vi "DP-Initialize Run.vi"(5 "Parameters":T1, 7 "acoustic system":string, 11 "error in (no error)":errorcluster) -> (4 "State":T4, 6 "DP Freqs":T5[](array[typedef]), 15 "error out":errorcluster)   [LabVIEW 2020]
uses:
  Typedefs/DP-Freqs.ctl
  Typedefs/DP-Runtime State.ctl
  Typedefs/DP-Parameters.ctl
  Typedefs/DP-Stimulus Params.ctl
  Typedefs/DP-Response Params.ctl
  9b327534-a05b-4f1e-8ea6-4dc0965c4c0a.vi
  53cc11d0-0777-45da-a4da-e21edc2e8946.vi
  0925d4c8-c7d7-466b-8d9d-3b6ad316888a.vi
  <vilib>/Utility/config.llb/Open Config Data.vi
  <vilib>/Utility/config.llb/Get Key Names.vi
  <vilib>/Utility/config.llb/Read Key.vi
  <vilib>/Utility/config.llb/Read Key (String).vi
  epl-vi-lib/Utility VIs/Array Manipulation VIs/String Array to Comma Separated String.vi
  <vilib>/Utility/error.llb/Error Cluster From Error Code.vi
  <vilib>/Utility/config.llb/Close Config Data.vi
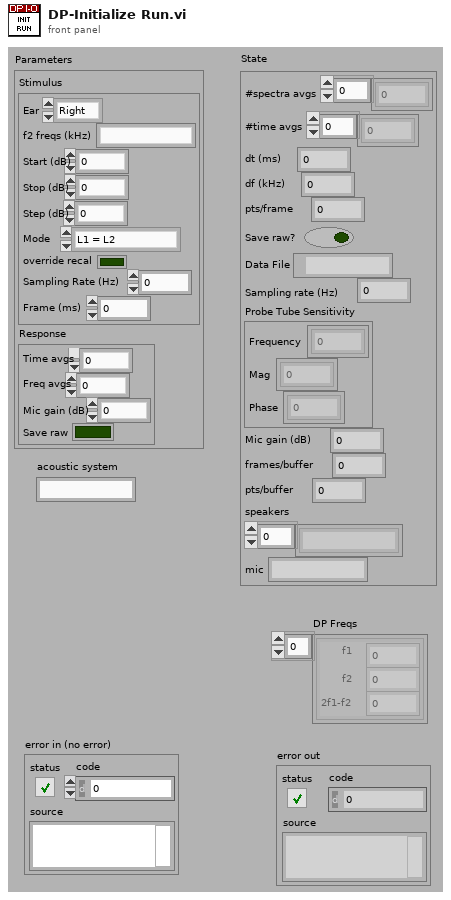
[diagram p1: front panel]
types:
  T1 = typedef "DP-Parameters.ctl" = cluster{"Stimulus":T2, "Response":T3}
  T2 = typedef "DP-Stimulus Params.ctl" = cluster{"Ear":enum16{"Right", "Left"}, "f2 freqs (kHz)":string, "Start (dB)":dbl, "Stop (dB)":dbl, "Step (dB)":dbl, "Mode":enum16{"L1 = L2", "L1 = L2 + 10 dB"}, "override recal":bool, "Sampling Rate (Hz)":dbl, "Frame (ms)":dbl}
  T3 = typedef "DP-Response Params.ctl" = cluster{"Time avgs":i32, "Freq avgs":i32, "Mic gain (dB)":dbl, "Save raw":bool}
  T4 = typedef "DP-Runtime State.ctl" = cluster{"#spectra avgs":i32[], "#time avgs":i32[], "dt (ms)":dbl, "df (kHz)":dbl, "pts/frame":i32, "Save raw?":bool, "Data File":path, "Sampling rate (Hz)":dbl, "Probe Tube Sensitivity":cluster{"Frequency":dbl[], "Mag":dbl[], "Phase":dbl[]}, "Mic gain (dB)":dbl, "frames/buffer":i32, "pts/buffer":i32, "speakers":string[], "mic":string}
  T5 = typedef "DP-Freqs.ctl" = cluster{"f1":dbl, "f2":dbl, "2f1-f2":dbl}
  T6 = cluster{"Coerced Frequency (kHz)":dbl, "Coerced Frequency (kHz)":dbl, dbl}
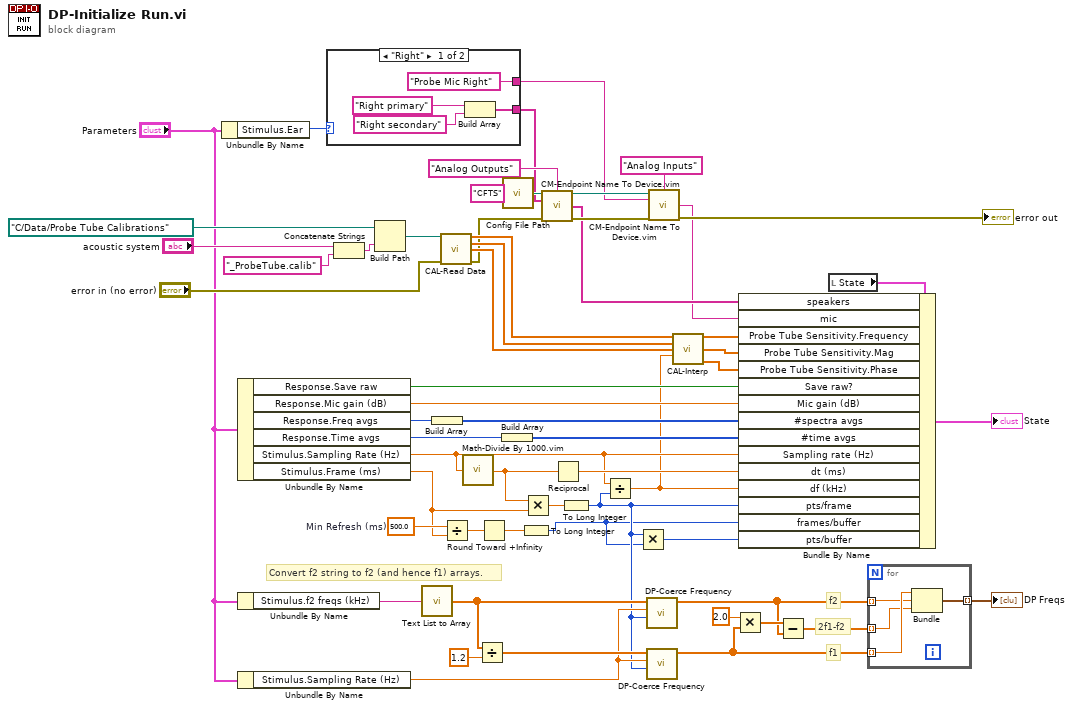
[diagram p0: block diagram]
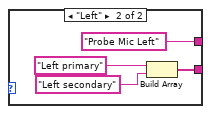
[diagram p2: hidden frame]
diagram:
  w28 = 500.0  # Min Refresh (ms)
  # "2f1-f2"
  # "f2"
  # "f1"
  # "Convert f2 string to f2 (and hence f1) arrays."
  n1 = Unbundle By Name("Parameters") -> ("Stimulus.Ear"=w14:enum16{"Right", "Left"})
  n2 = Unbundle By Name("Parameters") -> ("Response.Save raw"=w33:bool, "Response.Mic gain (dB)"=w34:dbl, "Response.Freq avgs"=w44:i32, "Response.Time avgs"=w43:i32, "Stimulus.Sampling Rate (Hz)"=w30:dbl, "Stimulus.Frame (ms)"=w27:dbl)
  n3 = Unbundle By Name("Parameters") -> ("Stimulus.f2 freqs (kHz)"=w56:string)
  n4 = Unbundle By Name("Parameters") -> ("Stimulus.Sampling Rate (Hz)"=w47:dbl)
  n5 = case shown="\"Right\"" w14 {
    tunnel: [w59 w63] -> w7
    tunnel: ["Probe Mic Right" "Probe Mic Left"] -> w8
    frame "Right" {
      n6 = Build Array("Right primary", "Right secondary") -> (w59:string[])
    }
    frame "Left" {
      n7 = Build Array("Left primary", "Left secondary") -> (w63:string[])
    }
  }
  n8 = Concatenate Strings("acoustic system", "_ProbeTube.calib") -> (w39:string)
  n9 = Build Path(base path=path "C:/Data/Probe Tube Calibrations", name or relative path=w39) -> (appended path=w35:path)
  n10 = call "Text List to Array.vi"("text list"=w56) -> ("array"=w55:dbl[])  [unwired: 3 in]
  n11 = Build Array(w44) -> (w41:i32[])
  n12 = call "CAL-Read Data.vi"("user path"=w35, "error in (no error)"="error in (no error)") -> ("Frequency (Hz)"=w18:dbl[], "Mag"=w17:dbl[], "Phase"=w16:dbl[], "error out"=w4:errorcluster)  [unwired: 9 in, 1 out]
  n13 = Divide(x=w28, y=w27) -> (x/y=w26:dbl)
  n14 = call "Math-Divide By 1000.vim"("X"=w30) -> ("1000X"=w32:dbl)
  n15 = Divide(x=w55, y=1.2) -> (x/y=w54:dbl[])
  n16 = Round Toward +Infinity(x=w26) -> (ceil(x): smallest int >= x=w25:dbl)
  n17 = Build Array(w43) -> (w40:i32[])
  n18 = call "Config File Path.vi"("AppName"="CFTS") -> ("Default config file name"=w12:path)
  n19 = To Long Integer(number=w25) -> (32bit integer=w23:i32)
  n20 = Multiply(x=w32, y=w27) -> (x*y=w31:dbl)
  n21 = call "CM-Endpoint Name To Device.vim"("Path"=w12, "IO Type"="Analog Outputs", "Names in"=w7, "error in (no error)"=w4) -> ("Path thru"=w9:path, "Devices"=w2:string[], "error out"=w6:errorcluster)  [unwired: 8 in, 1 out]
  n22 = Reciprocal(x=w32) -> (1/x=w42:dbl)
  n23 = To Long Integer(number=w31) -> (32bit integer=w24:i32)
  n24 = Divide(x=w30, y=w24) -> (x/y=w15:dbl)
  n25 = Multiply(x=w24, y=w23) -> (x*y=w22:i32)
  n26 = call "DP-Coerce Frequency.vi"("Npts"=w24, "Sampling rate (Hz)"=w47, "Frequency (kHz)"=w55) -> ("Coerced Frequency (kHz)"=w52:dbl[])  [unwired: 6 in, 2 out]
  n27 = call "DP-Coerce Frequency.vi"("Npts"=w24, "Sampling rate (Hz)"=w47, "Frequency (kHz)"=w54) -> ("Coerced Frequency (kHz)"=w50:dbl[])  [unwired: 6 in, 2 out]
  n28 = call "CM-Endpoint Name To Device.vim"("Path"=w9, "IO Type"="Analog Inputs", "Names in"=w8, "error in (no error)"=w6) -> ("Devices"=w1:string, "error out"=→"error out":errorcluster)  [unwired: 8 in, 2 out]
  n29 = call "CAL-Interp.vi"("Frequency (Hz)"=w18, "Magnitude (dB)"=w17, "Phase (degrees)"=w16, "df (Hz)"=w15) -> ("Interp Freq (Hz)"=w21:dbl[], "Interp Phase (degrees)"=w20:dbl[], "Interp z"=w19:cdb[])  [unwired: 8 in, 1 out]
  n30 = Multiply(x=2.0 ("y"), y=w50) -> (x*y=w53:dbl[])
  n31 = Subtract(x=w53, y=w52) -> (x-y=w49:dbl[])
  n32 = local read "State"() -> (w46:T4)
  n33 = Bundle By Name(cluster=w46, "speakers"=w2, "mic"=w1, "Probe Tube Sensitivity.Frequency"=w21, "Probe Tube Sensitivity.Mag"=w20, "Probe Tube Sensitivity.Phase"=w19, "Save raw?"=w33, "Mic gain (dB)"=w34, "#spectra avgs"=w41, "#time avgs"=w40, "Sampling rate (Hz)"=w30, "dt (ms)"=w42, "df (kHz)"=w15, "pts/frame"=w24, "frames/buffer"=w23, "pts/buffer"=w22) -> (→"State":T4)
  n34 = for {
    tunnel: w52 -> [w68] mode=indexing
    tunnel: w50 -> [w69] mode=indexing
    tunnel: w49 -> [w67] mode=indexing
    tunnel: [w66] -> w48 mode=indexing
    n35 = Bundle("Coerced Frequency (kHz)"=w69, "Coerced Frequency (kHz)"=w68, w67) -> (w66:T6)  [unwired: 1 in]
  }
  "DP Freqs" <- w48
